vi "Configure Generator Amplitude.vi"(0 "VISA resource name":refnum<visa-resource-name>, 1 "High Level (1.0 V)":dbl=1.0, 2 "Load Impendance (0: 1 MOhm)":i32(ring) items=["1 MOhm", "50 Ohm"], 5 "Setting Style (0: Amplitude + Offset)":i32(ring) items=["Amplitude + Offset", "High Level + Low Level"], 7 "Amplitude (1.0 V)":dbl=1.0, 9 "Offset (0.0 V)":dbl, 11 "error in (no error)":errorcluster, 12 "Low Level (0.0 V)":dbl, 13 "Waveform Generator Number (1: Waveform Generator 1)":i32(ring)=1 items=["Waveform Generator 1"=1, "Waveform Generator 2"=2]) -> (4 "VISA resource name out":refnum<visa-resource-name>, 15 "error out":errorcluster)   [LabVIEW 2023, in "Keysight-DSQx3014T.lvlib"]
doc: "Configures the waveform generator amplitude."
uses:
  Keysight-DSQx3014T.lvlib
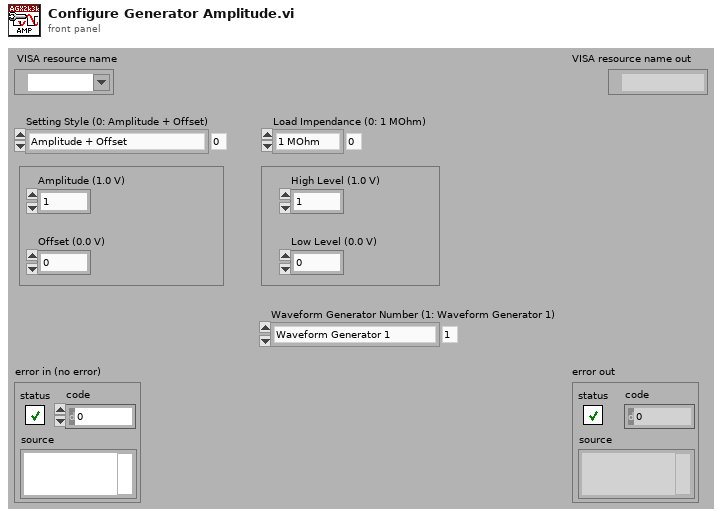
[diagram p1: front panel]
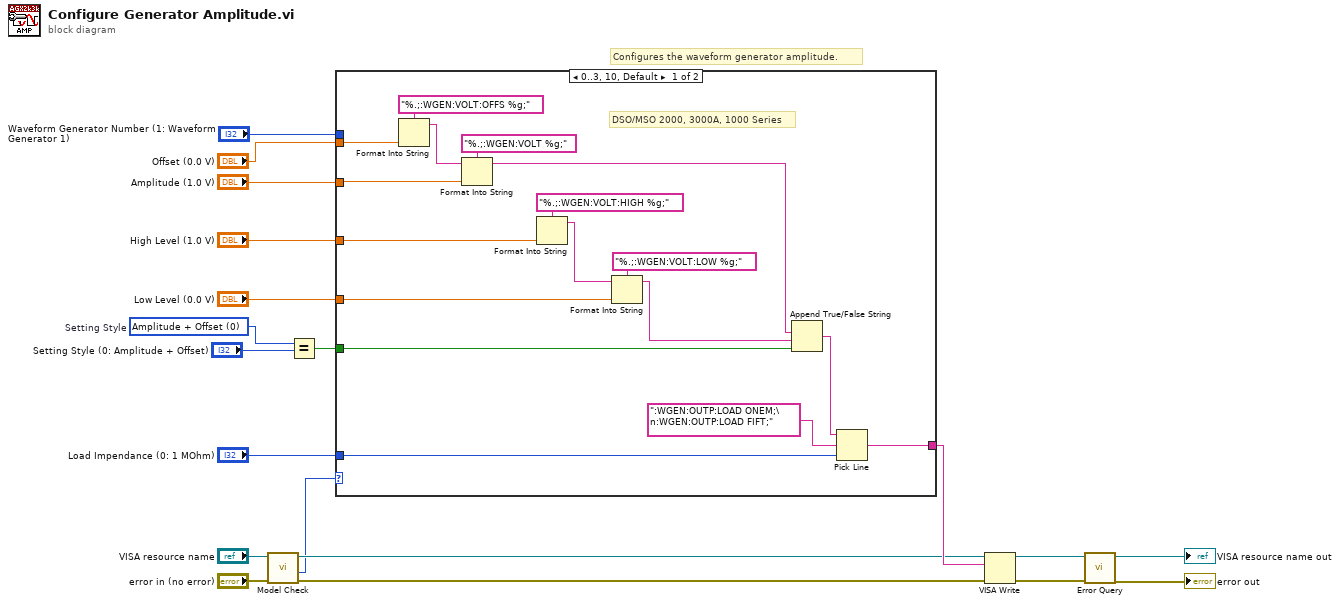
[diagram p0: block diagram]
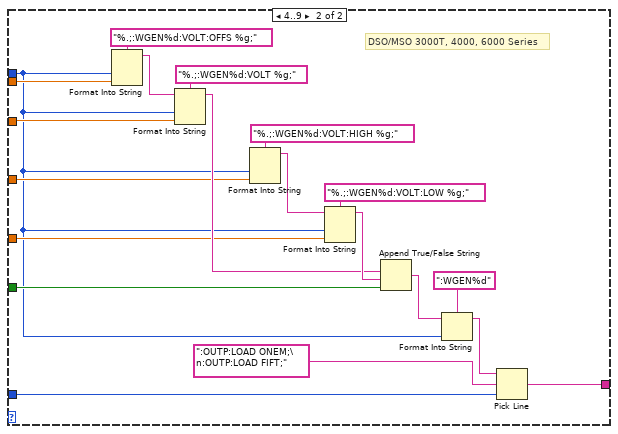
[diagram p2: hidden frame]
diagram:
  w9 = 0 items=["Amplitude + Offset", "High Level + Low Level"]  # Setting Style
  # "Configures the waveform generator amplitude."
  n1 = call "Model Check.vi"("error in (no error)"="error in (no error)", "VISA resource name"="VISA resource name") -> ("error out"=w2:errorcluster, "Model"=w1:i32, "VISA resource name out"=w3:refnum<visa-resource-name>)  [unwired: 7 out]
  n2 = Equal?(x=w9, y="Setting Style (0: Amplitude + Offset)") -> (x = y?=w7:bool)
  n3 = case shown="0..3, 10, Default" w1 {
    tunnel: "Amplitude (1.0 V)" -> [w35 w46]
    tunnel: "High Level (1.0 V)" -> [w33 w45]
    tunnel: "Low Level (0.0 V)" -> [w30 w44]
    tunnel: "Offset (0.0 V)" -> [w28 w47]
    tunnel: "Load Impendance (0: 1 MOhm)" -> [w26 w39]
    tunnel: [w25 w38] -> w14
    tunnel: w7 -> [w23 w43]
    tunnel: "Waveform Generator Number (1: Waveform Generator 1)" -> [_ w42]
    frame 0..3, 10, Default {
      # "DSO/MSO 2000, 3000A, 1000 Series"
      n4 = Format Into String(format string="%.;:WGEN:VOLT:OFFS %g;", w28) -> (resulting string=w24:string)  [unwired: 2 in, 1 out]
      n5 = Format Into String(format string="%.;:WGEN:VOLT %g;", initial string=w24, w35) -> (resulting string=w22:string)  [unwired: 1 in, 1 out]
      n6 = Format Into String(format string="%.;:WGEN:VOLT:HIGH %g;", w33) -> (resulting string=w32:string)  [unwired: 2 in, 1 out]
      n7 = Format Into String(format string="%.;:WGEN:VOLT:LOW %g;", initial string=w32, w30) -> (resulting string=w21:string)  [unwired: 1 in, 1 out]
      n8 = Append True/False String(1:w23, 2:w21, 3:w22) -> (0:w20:string)  [unwired: 1 out]
      n9 = Pick Line(string ("")=w20, multi-line string=":WGEN:OUTP:LOAD ONEM;\n:WGEN:OUTP:LOAD FIFT;", line index=w26) -> (output string=w25:string)
    }
    frame 4..9 {
      # "DSO/MSO 3000T, 4000, 6000 Series"
      n10 = Format Into String(format string="%.;:WGEN%d:VOLT:OFFS %g;", w42, w47) -> (resulting string=w54:string)  [unwired: 2 in, 1 out]
      n11 = Format Into String(format string="%.;:WGEN%d:VOLT %g;", initial string=w54, w42, w46) -> (resulting string=w55:string)  [unwired: 1 in, 1 out]
      n12 = Format Into String(format string="%.;:WGEN%d:VOLT:HIGH %g;", w42, w45) -> (resulting string=w50:string)  [unwired: 2 in, 1 out]
      n13 = Format Into String(format string="%.;:WGEN%d:VOLT:LOW %g;", initial string=w50, w42, w44) -> (resulting string=w56:string)  [unwired: 1 in, 1 out]
      n14 = Append True/False String(1:w43, 2:w56, 3:w55) -> (0:w41:string)  [unwired: 1 out]
      n15 = Format Into String(format string=":WGEN%d", initial string=w41, w42) -> (resulting string=w40:string)  [unwired: 1 in, 1 out]
      n16 = Pick Line(string ("")=w40, multi-line string=":OUTP:LOAD ONEM;\n:OUTP:LOAD FIFT;", line index=w39) -> (output string=w38:string)
    }
  }
  n17 = VISA Write(VISA resource name=w3, write buffer=w14, error in (no error)=w2) -> (VISA resource name out=w13:refnum<visa-resource-name>, error out=w12:errorcluster)  [unwired: 1 out]
  n18 = call "Error Query.vi"("error in (no error)"=w12, "VISA resource name"=w13) -> ("error out"=→"error out":errorcluster, "VISA resource name out"=→"VISA resource name out":refnum<visa-resource-name>)  [unwired: 8 out]
